vi "Publish.vi"(0 "Topic":string="/junk", 1 "node":string, 2 "String":string, 3 "error in":errorcluster) -> (7 "error":errorcluster)   [LabVIEW 2012]
doc: "Starts a publisher on the RIO"
uses:
  <userlib>/ROS for LabVIEW Software/ROS/Code/Console/Servers/ServerSubs/TopicDef.ctl
  <userlib>/ROS for LabVIEW Software/ROS/Code/SubVIs/_ROSDirection.ctl
  <userlib>/ROS for LabVIEW Software/ROS/MessageBuilding/std_msgs/subs/stringScalar.vi
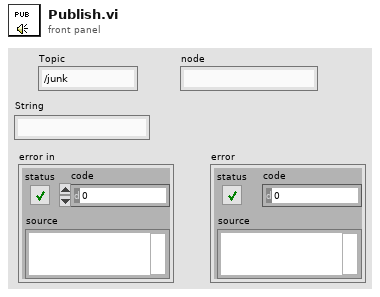
[diagram p1: front panel]
types:
  T1 = typedef "TopicDef.ctl" = cluster{"Topic":string, "Type":string, "Action":T2, "Update (ms)":u16, "queue size":u16}
  T2 = typedef "_ROSDirection.ctl" = enum16{"Node", "Publisher", "Subscriber", "ServiceClient", "ServiceProvider"}
  T3 = typedef "_ROSControl.ctl" = cluster{"topic port":u16, "Node":string, "topic":string, "type":string, "node port":u16, "error ":errorcluster, "Direction":T2, "Update (ms)":u16, "FIFO size":u16}
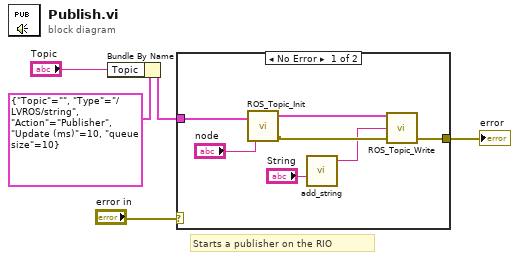
[diagram p0: block diagram]
diagram:
  # "Starts a publisher on the RIO"
  n1 = Bundle By Name(cluster=T1 {"Topic"="", "Type"="/LVROS/string", "Action"=enum."Publisher", "Update (ms)"=10, "queue size"=10} ("Definitions"), "Topic"="Topic") -> (w4:T1)
  n2 = case shown="No Error" "error in" {
    selector: "error in" -> [_ w13]
    tunnel: w4 -> [w9 _]
    tunnel: [w8 w13] -> w2
    frame No Error {
      n3 = call <userlib>:"ROS_Topic_Init.vi"("Definitions"=w9, "node"="node") -> ("ROS out"=w12:T3, "error out"=w7:errorcluster)  [unwired: 1 in]
      n4 = call-poly <userlib>:"add_string.vi"("String"="String") -> ("msg out"=w6:string)  [unwired: 4 in]
      n5 = call <userlib>:"ROS_Topic_Write.vi"("error in (no error)"=w7, "Msg in"=w6, "ROS in"=w12) -> ("error out"=w8:errorcluster)  [unwired: 1 in, 1 out]
    }
    frame Error {
    }
  }
  "error" <- w2
